vi "[GUIDELINE]ReadFromDashboard.vi"() -> (14 "boolCalData":bool[](array[boolean]), 15 "boolCalDataNames":string[](array[string]), 16 "numCalData":dbl[](array[numeric]), 17 "numCalDataNames":string[](array[string]), 18 "stringCalData":string[](array[string]), 19 "stringCalDataNames":string[](array[string]))   [LabVIEW 2020]
uses:
  <vilib>/Rock Robotics/WPI/DriverStation/WPI_DriverStationRobotMode2.ctl
  <vilib>/Rock Robotics/Network Tables/NT Read Boolean Array.vi
  <vilib>/Rock Robotics/Network Tables/NT Read String Array.vi
  <vilib>/Rock Robotics/Network Tables/NT Read Numeric Array.vi
  2021-MARS-Swerve/Robot Global Data.vi
  2021-MARS-Swerve/Globals/Magazine_Globals.vi
  2021-MARS-Swerve/Globals/Intake_Globals.vi
  2021-MARS-Swerve/Globals/Sensor_Values.vi
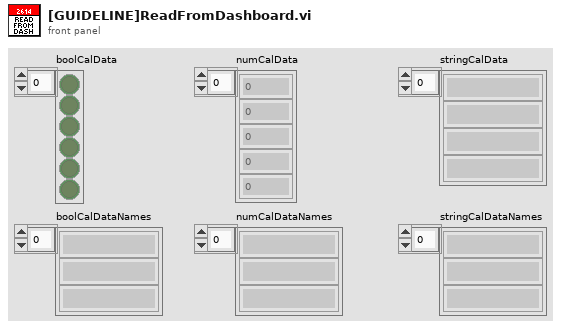
[diagram p1: front panel]
types:
  T1 = typedef "WPI_DriverStationRobotMode2.ctl" = enum16{"Autonomous Disabled", "Autonomous Enabled", "Teleop Disabled", "Teleop Enabled", "Disconnected", "Finish", "Test Disabled", "Test Enabled", "Emergency Stopped"}
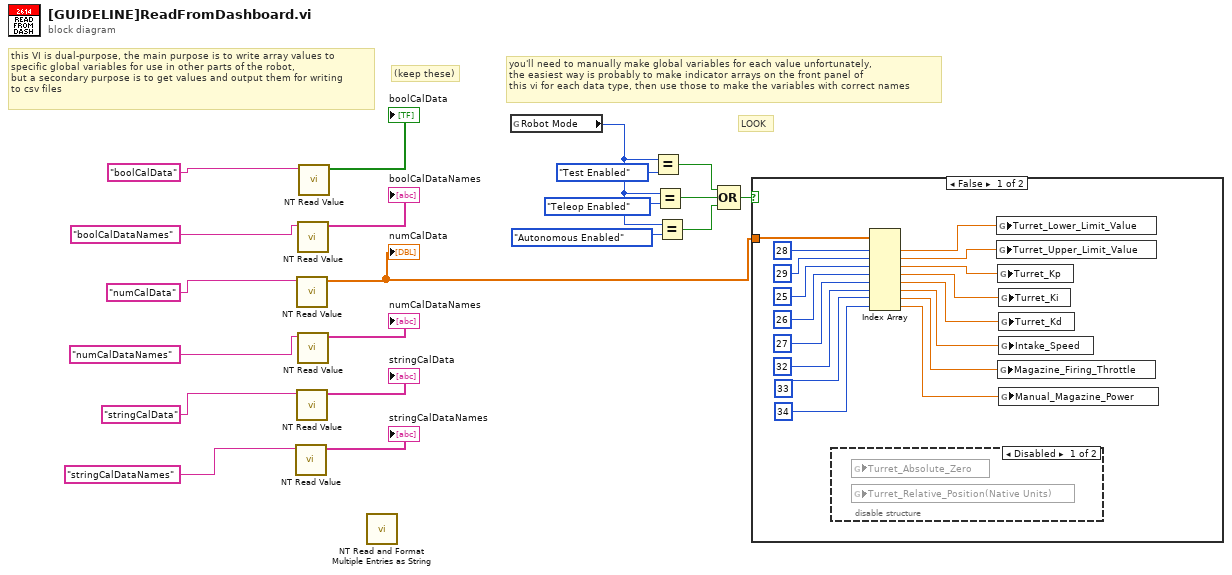
[diagram p0: block diagram]
diagram:
  # "(keep these)"
  # "this VI is dual-purpose, the main purpose is to write array values to \nspecific global variables for use in other parts of the robot, \nbut a secondary purpose is to get values and output them for writing\nto csv files"
  # "LOOK"
  # "you'll need to manually make global variables for each value unfortunately,\nthe easiest way is probably to make indicator arrays on the front panel of\nthis vi for each data type, then use those to make the variables with correct names"
  n1 = call-poly <vilib>:"NT Read Value.vi"("Name"="stringCalDataNames" ("stringCalDataNames")) -> ("String Array"=→"stringCalDataNames":string[])  [unwired: 9 in, 1 out]
  n2 = call-poly <vilib>:"NT Read Value.vi"("Name"="numCalData" ("numCalData")) -> ("Numeric Array"=w1:dbl[])  [unwired: 9 in, 1 out]
  "numCalData" <- w1
  n3 = call-poly <vilib>:"NT Read Value.vi"("Name"="stringCalData" ("stringCalData")) -> ("String Array"=→"stringCalData":string[])  [unwired: 9 in, 1 out]
  n4 = call-poly <vilib>:"NT Read Value.vi"("Name"="boolCalDataNames" ("boolCalDataNames")) -> ("String Array"=→"boolCalDataNames":string[])  [unwired: 9 in, 1 out]
  n5 = call-poly <vilib>:"NT Read Value.vi"("Name"="numCalDataNames" ("numCalDataNames")) -> ("String Array"=→"numCalDataNames":string[])  [unwired: 9 in, 1 out]
  n6 = call-poly <vilib>:"NT Read Value.vi"("Name"="boolCalData" ("boolCalData")) -> ("Boolean Array"=→"boolCalData":bool[])  [unwired: 9 in, 1 out]
  n7 = call <vilib>:"NT Read and Format Multiple Entries as String.vi"() -> ()  [unwired: 10 in, 2 out]
  n8 = global read "Robot Global Data.vi" "Robot Mode"() -> (w2:T1)
  n9 = Equal?(x=w2, y=WPI_DriverStationRobotMode2."Test Enabled") -> (x = y?=w7:bool)
  n10 = Equal?(x=w2, y=WPI_DriverStationRobotMode2."Teleop Enabled") -> (x = y?=w6:bool)
  n11 = Equal?(x=w2, y=WPI_DriverStationRobotMode2."Autonomous Enabled") -> (x = y?=w5:bool)
  n12 = Compound Arithmetic op=OR(w7, w6, w5) -> (w4:bool)
  n13 = case shown="False" w4 {
    tunnel: w1 -> [w37 _]
    frame False {
      n14 = disable-structure shown="Disabled" {
        frame Disabled {
          n15 = global read "Sensor_Values.vi" "Turret_Absolute_Zero"() -> ()  [unwired: 1 in]
          n16 = global read "Sensor_Values.vi" "Turret_Relative_Position(Native Units)"() -> ()  [unwired: 1 in]
        }
        frame Enabled {
        }
      }
      n17 = Index Array(array=w37, index #1=28 ("index"), index #2=29 ("index"), index #3=25 ("index"), index #4=26 ("index"), index #5=27 ("index"), index #6=32 ("index"), index #7=33 ("index"), index #8=34 ("index")) -> (element #1=w36:dbl, element #2=w35:dbl, element #3=w32:dbl, element #4=w31:dbl, element #5=w30:dbl, element #6=w26:dbl, element #7=w25:dbl, element #8=w22:dbl)
      n18 = global write "Sensor_Values.vi" "Turret_Lower_Limit_Value"(w36) -> ()
      n19 = global write "Sensor_Values.vi" "Turret_Upper_Limit_Value"(w35) -> ()
      n20 = global write "Sensor_Values.vi" "Turret_Kp"(w32) -> ()
      n21 = global write "Magazine_Globals.vi" "Magazine_Firing_Throttle"(w25) -> ()
      n22 = global write "Sensor_Values.vi" "Turret_Ki"(w31) -> ()
      n23 = global write "Sensor_Values.vi" "Turret_Kd"(w30) -> ()
      n24 = global write "Intake_Globals.vi" "Intake_Speed"(w26) -> ()
      n25 = global write "Magazine_Globals.vi" "Manual_Magazine_Power"(w22) -> ()
    }
    frame True {
      # "nothing is written"
    }
  }
